vi "test_distance.vi"() -> ()   [LabVIEW 2019]
panel:
  out "out":dbl
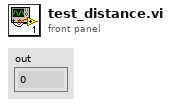
[diagram p1: front panel]
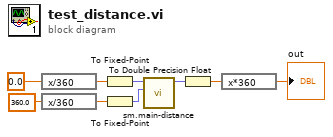
[diagram p0: block diagram]
diagram:
  n1 = expression code="x/360"(0.0) -> (w7:dbl)
  n2 = expression code="x/360"(360.0) -> (w6:dbl)
  n3 = To Fixed-Point(number=w7) -> (fixed-point=w4:fxp<+/-,32,2>)  [unwired: 1 in]
  n4 = To Fixed-Point(number=w6) -> (fixed-point=w5:fxp<+/-,32,2>)  [unwired: 1 in]
  n5 = call "sm.main-distance.vi"("y"=w5, "x"=w4) -> ("distance"=w3:fxp<+/-,32,2>)  [unwired: 9 in]
  n6 = To Double Precision Float(number=w3) -> (double precision float=w2:dbl)
  n7 = expression code="x*360"(w2) -> (→"out":dbl)
